vi "CMD_SETDISPENSE.vi"(6 "Gantry in":refnum<class "Gantry.lvclass">, 8 "error in (no error)":errorcluster, 10 "Arguments":string[](array[string]), 11 "gScript Interpreter in":refnum<class "gScript Interpreter.lvclass">) -> (0 "error out":errorcluster, 3 "gScript Interpreter out":refnum<class "gScript Interpreter.lvclass">, 4 "Gantry out":refnum<class "Gantry.lvclass">)   [LabVIEW 2024, in "gScript Interpreter.lvclass"]
uses:
  gScript Interpreter.lvclass
  Shared Components/Gantry Class/Gantry.lvclass
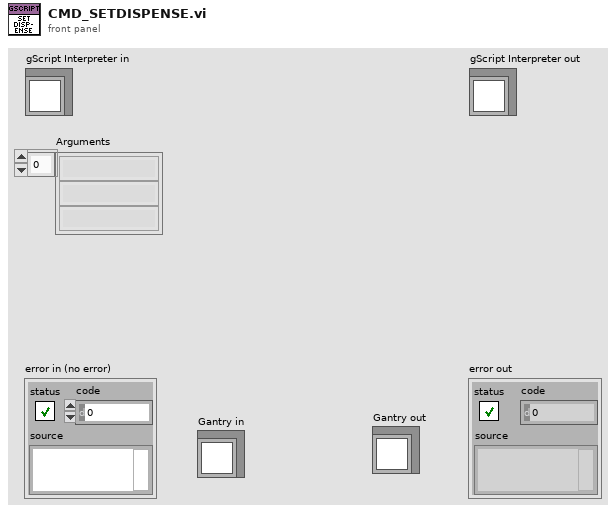
[diagram p1: front panel]
types:
  T1 = typedef "Memory Cell.ctl" = cluster{"type":T2, "x":dbl, "y":dbl, "z":dbl, "w":dbl}
  T2 = typedef "Memory Cell Type Enum.ctl" = enum16{"integer", "float", "vector", "rotation"}
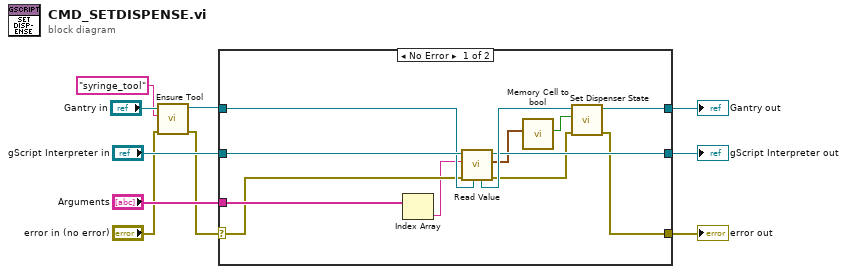
[diagram p0: block diagram]
diagram:
  n1 = call "Ensure Tool.vi"("error in (no error)"="error in (no error)", "Tool Name"="syringe_tool", "Gantry in"="Gantry in") -> ("error out"=w2:errorcluster, "Gantry out"=w4:refnum<class "Gantry.lvclass">)  [unwired: 7 in]
  n2 = case shown="No Error" w2 {
    selector: w2 -> [w17 w25]
    tunnel: [w11 w25] -> w10
    tunnel: [w15 w24] -> w8
    tunnel: "gScript Interpreter in" -> [w20 w24]
    tunnel: "Arguments" -> [w22 _]
    tunnel: w4 -> [w19 w23]
    tunnel: [w21 w23] -> w5
    frame No Error {
      n3 = Index Array(array=w22) -> (element=w16:string)  [unwired: 1 in]
      n4 = call-dynamic "Read Value.vi"("Gantry in"=w19, "error in (no error)"=w17, "String in"=w16, "gScript Interpreter in"=w20) -> ("error out"=w12:errorcluster, "Memory Cell"=w14:T1, "gScript Interpreter out"=w15:refnum<class "gScript Interpreter.lvclass">, "Gantry out"=w18:refnum<class "Gantry.lvclass">)  [unwired: 4 in]
      n5 = call "Memory Cell to bool.vi"("Memory Cell"=w14) -> ("bool out"=w13:bool)  [unwired: 10 in]
      n6 = call-dynamic "Set Dispenser State.vi"("error in"=w12, "On/Off"=w13, "Gantry in"=w18) -> ("error out"=w11:errorcluster, "Gantry out"=w21:refnum<class "Gantry.lvclass">)  [unwired: 7 in]
    }
    frame Error {
    }
  }
  "error out" <- w10
  "gScript Interpreter out" <- w8
  "Gantry out" <- w5
